vi "Write Grabbed Tool.vi"(8 "error in (no error)":errorcluster, 10 "Grabbed Tool":enum16{"Weight Tool", "Stamp Tool", "Nothing"}(ring)=enum."Nothing", 11 "GrabberTool Class in":refnum<class "GrabberTool Class.lvclass">) -> (0 "error out":errorcluster, 3 "GrabberTool Class out":refnum<class "GrabberTool Class.lvclass">)   [LabVIEW 2011, in "GrabberTool Class.lvclass"]
uses:
  GrabberTool Class.lvclass
  GrabberTool Class.lvclass/GrabberTool Class.ctl
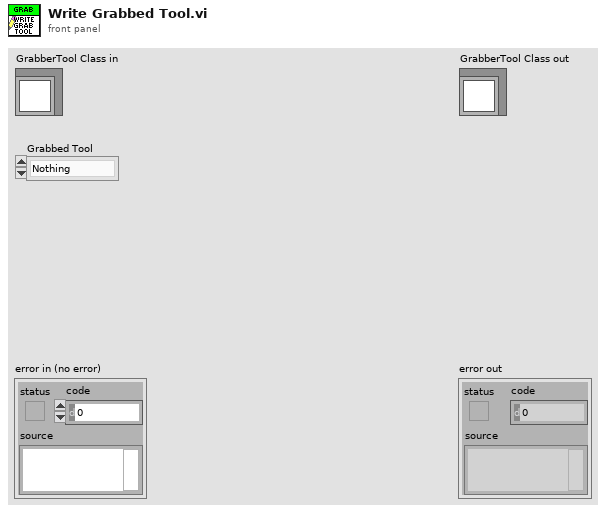
[diagram p1: front panel]
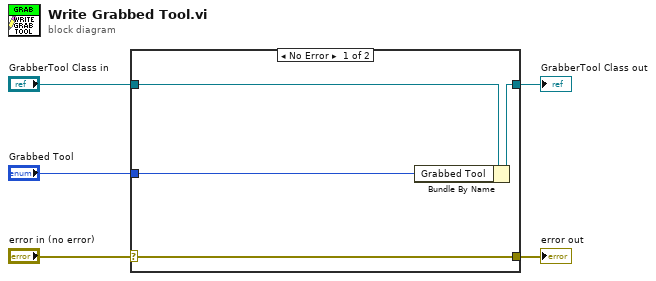
[diagram p0: block diagram]
diagram:
  n1 = case shown="No Error" "error in (no error)" {
    selector: "error in (no error)" -> [w9 w10]
    tunnel: [w9 w10] -> w4
    tunnel: [w7 w11] -> w2
    tunnel: "GrabberTool Class in" -> [w8 w11]
    tunnel: "Grabbed Tool" -> [w6 _]
    frame No Error {
      n2 = Bundle By Name(cluster=w8, "Grabbed Tool"=w6) -> (w7:refnum<class "GrabberTool Class.lvclass">)
    }
    frame Error {
    }
  }
  "error out" <- w4
  "GrabberTool Class out" <- w2
